vi "Fpga-Last-NonZeroValue-U64.vi"(11 "d_mcs_i\\IO_BUS_write_data in":u64) -> (3 "d_mcs_i\\IO_BUS_write_data out":u64)   [LabVIEW 2017]
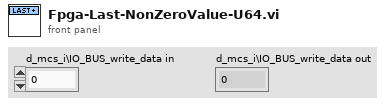
[diagram p1: front panel]
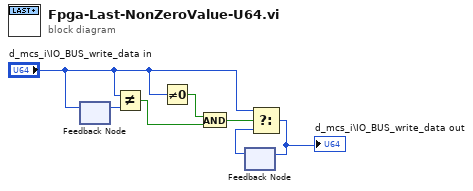
[diagram p0: block diagram]
diagram:
  n1 = feedback #1() -> (w1:u64)  [unwired: 1 in]
  n2 = feedback-in #1("d_mcs_i\\IO_BUS_write_data in") -> ()
  n3 = Not Equal?(x="d_mcs_i\\IO_BUS_write_data in", y=w1) -> (x != y?=w2:bool)
  n4 = Not Equal To 0?(x="d_mcs_i\\IO_BUS_write_data in") -> (x != 0?=w3:bool)
  n5 = And(x=w3, y=w2) -> (x .and. y?=w4:bool)
  n6 = feedback #2() -> (w7:u64)  [unwired: 1 in]
  n7 = Select(t="d_mcs_i\\IO_BUS_write_data in", s=w4, f=w7) -> (s? t:f=w6:u64)
  "d_mcs_i\\IO_BUS_write_data out" <- w6
  n8 = feedback-in #2(w6) -> ()
